vi "Delay.vi"(8 "error in":errorcluster, 10 "delay(ms)":u32) -> (0 "error out":errorcluster)   [LabVIEW 2012]
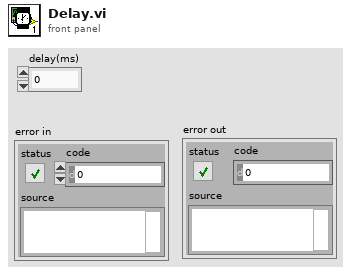
[diagram p1: front panel]
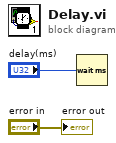
[diagram p0: block diagram]
diagram:
  n1 = Wait (ms)(milliseconds to wait="delay(ms)") -> ()  [unwired: 1 out]
  "error out" <- "error in"
